vi "ChangeStaticVoltage.vi"(8 "Channel to change":i32, 9 "Voltage":dbl, 10 "Parameters input":T2) -> (1 "Voltage out":dbl, 2 "Parameters Output":T2)   [LabVIEW 2013]
uses:
  6704/6704_static_voltages_control.ctl
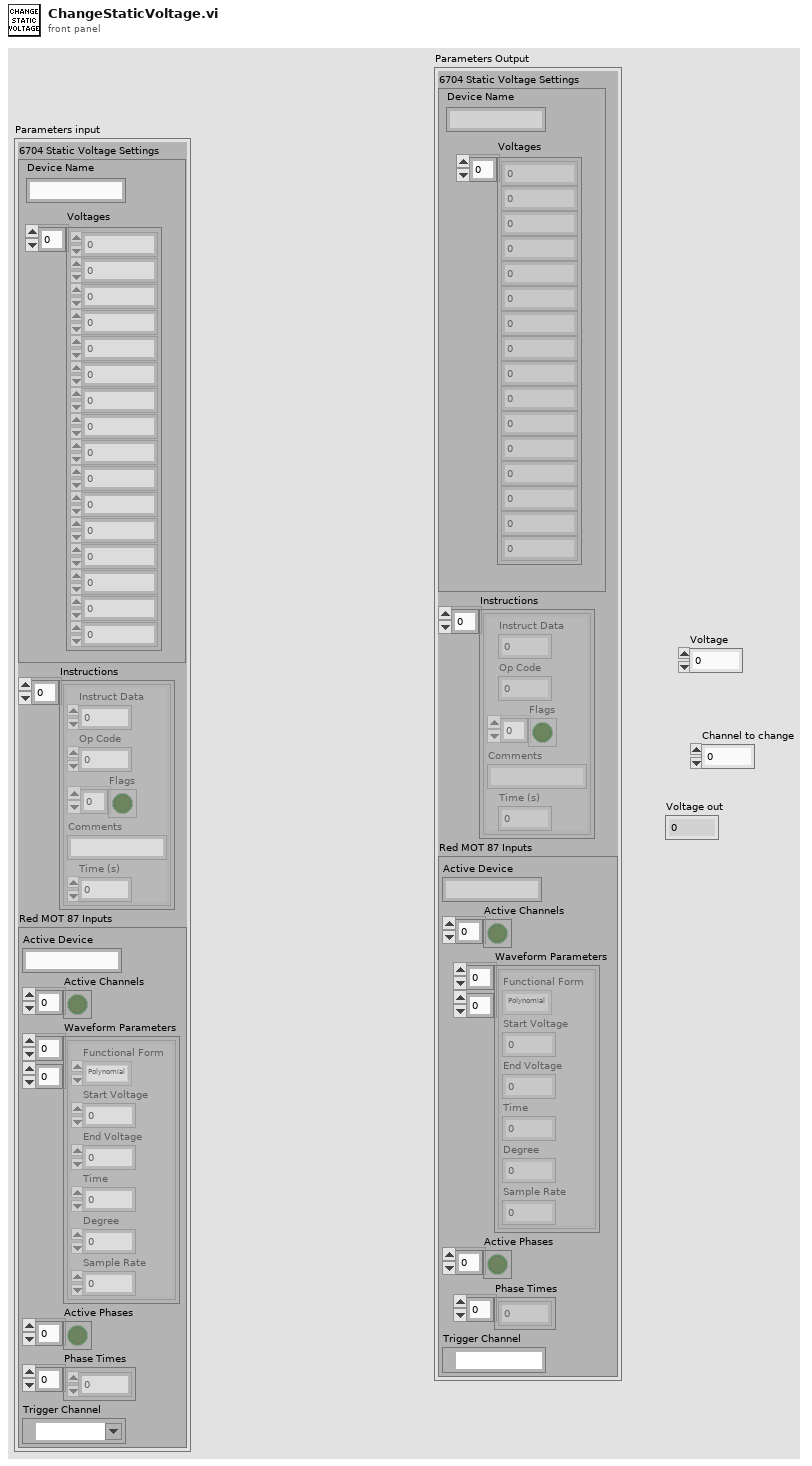
[diagram p1: front panel]
types:
  T1 = typedef "6704_static_voltages_control.ctl" = cluster{"Device Name":string, "Voltages":dbl[]}
  T2 = cluster{"6704 Static Voltage Settings":T1, "Instructions":cluster{"Instruct Data":i32, "Op Code":i32, "Flags":bool[], "Comments":string, "Time (s)":dbl}[], "Red MOT 87 Inputs":cluster{"Active Device":string, "Active Channels":bool[], "Waveform Parameters":cluster{"Functional Form":enum16{"Polynomial", "Exponential"}, "Start Voltage":dbl, "End Voltage":dbl, "Time":dbl, "Degree":i8, "Sample Rate":dbl}[][], "Active Phases":bool[], "Phase Times":dbl[], "Trigger Channel":tag}}
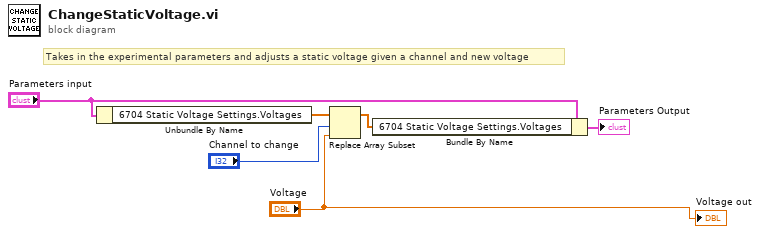
[diagram p0: block diagram]
diagram:
  # "Takes in the experimental parameters and adjusts a static voltage given a channel and new voltage"
  n1 = Unbundle By Name("Parameters input") -> ("6704 Static Voltage Settings.Voltages"=w5:dbl[])
  n2 = Replace Array Subset(array=w5, new element="Voltage", index="Channel to change") -> (w3:dbl[])
  n3 = Bundle By Name(cluster="Parameters input", "6704 Static Voltage Settings.Voltages"=w3) -> (→"Parameters Output":T2)
  "Voltage out" <- "Voltage"
